vi "Circle.vi"(6 "Fill Color":u32(colorbox), 7 "fill?(F)":bool, 8 "error in (no error)":errorcluster, 9 "Edge Color":u32(colorbox), 10 "rect":T1, 11 "Tools Paint in":refnum<class "Tools Paint.lvclass">) -> (0 "error out":errorcluster, 2 "new picture":picture, 3 "Tools Paint out":refnum<class "Tools Paint.lvclass">)   [LabVIEW 2021, in "Tools Paint.lvclass"]
uses:
  <resource>/plugins/NIIconEditor/Class/Tools/Tools Paint.lvclass
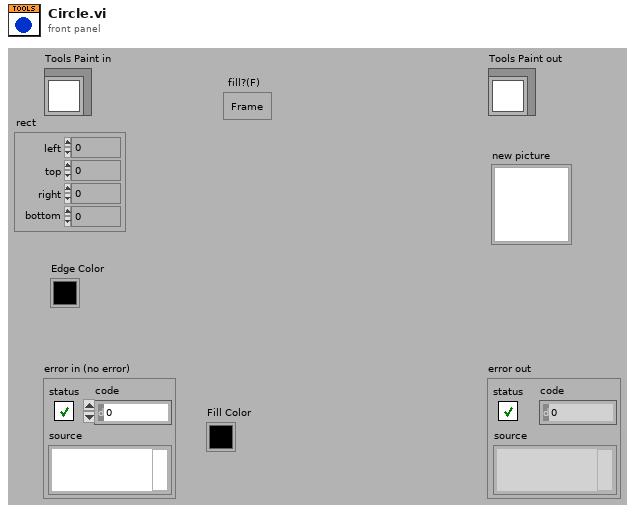
[diagram p1: front panel]
types:
  T1 = cluster{"left":i16, "top":i16, "right":i16, "bottom":i16}
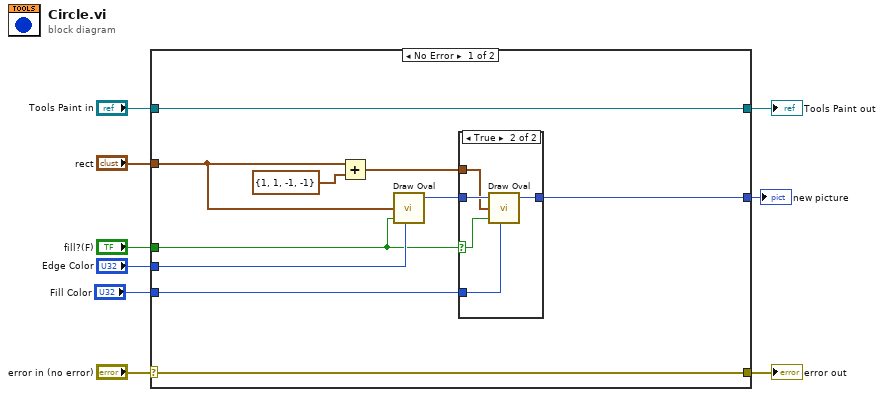
[diagram p0: block diagram]
diagram:
  n1 = case shown="No Error" "error in (no error)" {
    selector: "error in (no error)" -> [w18 w27]
    tunnel: [w18 w27] -> w8
    tunnel: [w19 w26] -> w6
    tunnel: "Tools Paint in" -> [w19 w26]
    tunnel: [w14 _] -> w5
    tunnel: "rect" -> [w12 _]
    tunnel: "fill?(F)" -> [w16 _]
    tunnel: "Edge Color" -> [w17 _]
    tunnel: "Fill Color" -> [w13 _]
    frame No Error {
      n2 = Add(x=w12, y=T1 {"left"=1, "top"=1, "right"=-1, "bottom"=-1}) -> (x+y=w10:T1)
      n3 = call <vilib>:"Draw Oval.vi"("rect"=w12, "fill?(F)"=w16, "color(black)"=w17) -> ("new picture"=w15:picture)  [unwired: 2 in, 4 out]
      n4 = case shown="True" w16 {
        selector: w16 -> [_ w21]
        tunnel: w15 -> [w20 w25]
        tunnel: [w20 w24] -> w14
        tunnel: w13 -> [_ w23]
        tunnel: w10 -> [_ w22]
        frame False {
        }
        frame True {
          n5 = call <vilib>:"Draw Oval.vi"("picture"=w25, "rect"=w22, "fill?(F)"=w21, "color(black)"=w23) -> ("new picture"=w24:picture)  [unwired: 1 in, 4 out]
        }
      }
    }
    frame Error {
    }
  }
  "error out" <- w8
  "Tools Paint out" <- w6
  "new picture" <- w5
